vi "Is Error Case.vi"(8 "error in (no error)":errorcluster, 11 "variant":variant) -> (0 "error out":errorcluster, 3 "error cluster?":bool)   [LabVIEW 2017]
uses:
  <vilib>/Utility/Data Type/Type Definitions/Data Type.ctl
  <vilib>/Utility/Data Type/NI_Data Type.lvlib
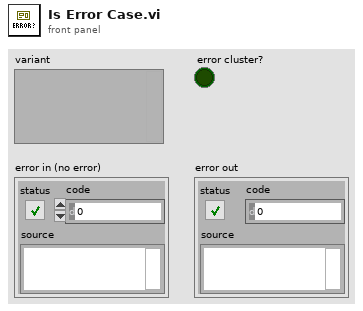
[diagram p1: front panel]
types:
  T1 = typedef "NI_Data Type.lvlib/Data Type.ctl" = enum8{"Invalid Type", "Void", "I8", "I16", "I32", "I64", "U8", "U16", "U32", "U64", "Single Float", "Double Float", "Extended Float", "Single Complex", "Double Complex", "Extended Complex", "Enum U8", "Enum U16", "Enum U32", "Enum U64", "Single Float With Unit", "Double Float With Unit", "Extended Float With Unit", "Single Complex with Unit", "Double Complex with Unit", "Extended Complex with Unit", "Boolean", "String", "Path", "Picture", "Tag", "Array", "Cluster", "Variant", "LV Variant", "Waveform", "Timestamp", "Digital Waveform", "Digital Data", "ExpressData", "Refnum", "External Data", "VI", "Poly VI", "LabVIEW Class Instance", "Fixed Point"}
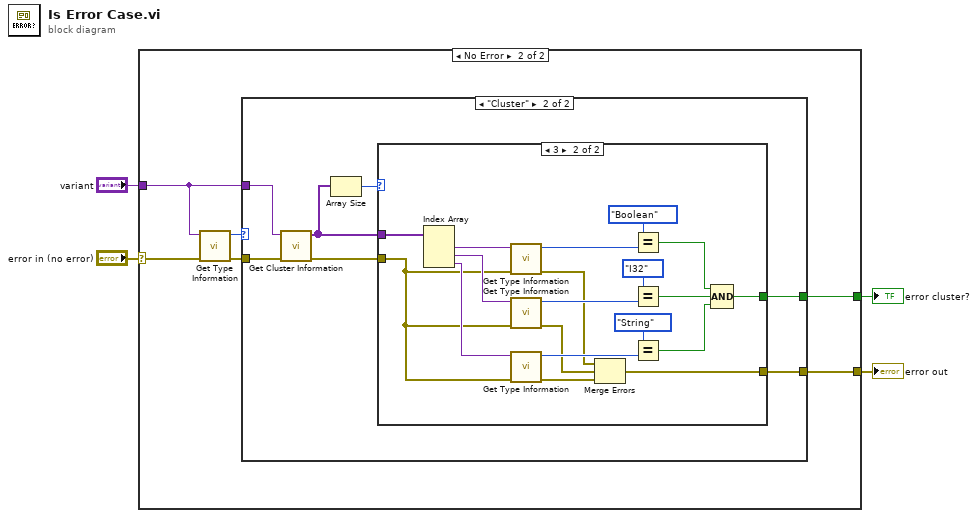
[diagram p0: block diagram]
diagram:
  n1 = case shown="No Error" "error in (no error)" {
    selector: "error in (no error)" -> [w5 w7]
    tunnel: "variant" -> [_ w9]
    tunnel: [w5 w8] -> w2
    tunnel: [_ w6] -> w1
    frame Error {
    }
    frame No Error {
      n2 = call <vilib>:"Get Type Information.vi"("error in (no error)"=w7, "Variant"=w9) -> ("error out"=w10:errorcluster, "Type"=w11:T1)  [unwired: 5 in, 3 out]
      n3 = case shown="\"Cluster\"" w11 {
        tunnel: w10 -> [w12 w19]
        tunnel: w9 -> [_ w18]
        tunnel: [w12 w14] -> w8
        tunnel: [_ w13] -> w6
        frame Default {
        }
        frame "Cluster" {
          n4 = call <vilib>:"Get Cluster Information.vi"("error in (no error)"=w19, "Variant"=w18) -> ("error out"=w15:errorcluster, "Cluster Elements"=w16:variant[])  [unwired: 8 in]
          n5 = Array Size(array=w16) -> (size(s)=w17:i32)
          n6 = case shown="3" w17 {
            tunnel: w16 -> [_ w39]
            tunnel: w15 -> [w20 w35]
            tunnel: [_ w22] -> w13
            tunnel: [w20 w21] -> w14
            frame Default {
            }
            frame 3 {
              n7 = Index Array(array=w39) -> (element #1=w38:variant, element #2=w37:variant, element #3=w36:variant)  [unwired: 3 in]
              n8 = call <vilib>:"Get Type Information.vi"("error in (no error)"=w35, "Variant"=w38) -> ("error out"=w28:errorcluster, "Type"=w34:T1)  [unwired: 5 in, 3 out]
              n9 = call <vilib>:"Get Type Information.vi"("error in (no error)"=w35, "Variant"=w37) -> ("error out"=w27:errorcluster, "Type"=w31:T1)  [unwired: 5 in, 3 out]
              n10 = call <vilib>:"Get Type Information.vi"("error in (no error)"=w35, "Variant"=w36) -> ("error out"=w26:errorcluster, "Type"=w29:T1)  [unwired: 5 in, 3 out]
              n11 = Merge Errors(w28, w27, w26) -> (w21:errorcluster)
              n12 = Equal?(x=Data_Type."Boolean", y=w34) -> (x = y?=w25:bool)
              n13 = Equal?(x=Data_Type."I32", y=w31) -> (x = y?=w24:bool)
              n14 = Equal?(x=Data_Type."String", y=w29) -> (x = y?=w23:bool)
              n15 = Compound Arithmetic op=AND(w25, w24, w23) -> (w22:bool)
            }
          }
        }
      }
    }
  }
  "error out" <- w2
  "error cluster?" <- w1
